vi "Impulse Response Function PtByPt.vi"(2 "initialize":bool, 3 "sample length":i32=100, 4 "response signal y":dbl format="%0.2f", 5 "stimulus signal x":dbl format="%0.2f") -> (0 "error":i32, 1 "Impulse Response":dbl[](array[numeric]))   [LabVIEW 2017, in "NI_PtbyPt.lvlib"]
doc: "Computes the impulse response of a network based on the set of real signals x, <B>stimulus signal x</B>, and y, <B>response signal y</B>."
uses:
  <vilib>/ptbypt/NI_PtbyPt.lvlib
  <vilib>/Analysis/2dsp.llb/Inverse Real FFT.vi
  <vilib>/Analysis/NI_AALPro.lvlib
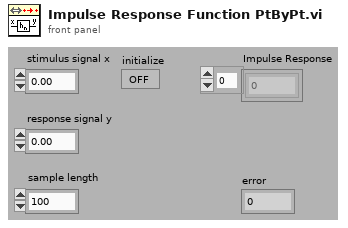
[diagram p1: front panel]
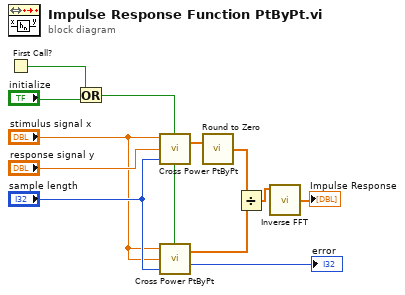
[diagram p0: block diagram]
diagram:
  n1 = First Call?() -> (First Call?: T/F=w1:bool)
  n2 = Or(x=w1, y="initialize") -> (x .or. y?=w3:bool)
  n3 = call <vilib>:"Cross Power PtByPt.vi"("initialize"=w3, "sample length"="sample length", "y"="response signal y", "x"="stimulus signal x") -> ("Sxy"=w7:cdb[])  [unwired: 1 out]
  n4 = call <vilib>:"Cross Power PtByPt.vi"("initialize"=w3, "sample length"="sample length", "y"="stimulus signal x", "x"="stimulus signal x") -> ("error"=→"error":i32, "Sxy"=w4:cdb[])
  n5 = call <vilib>:"Round to Zero.vi"("complex"=w7) -> ("result"=w6:cdb[])
  n6 = Divide(x=w6, y=w4) -> (x/y=w11:cdb[])
  n7 = call-poly <vilib>:"Inverse FFT.vi"("FFT {X}"=w11) -> ("X"=→"Impulse Response":dbl[])  [unwired: 9 in, 1 out]
